vi "LensDistortionCorrectionRpiCam.vi"() -> ()   [LabVIEW 2019]
panel:
  out "Image 2":T1(plugin-control)
  out "Image":T1(plugin-control)
  in  "File Path (Image Calibration 1)":path=path "C:/Users/TTUHEP/Pictures/CalibratedrPiImage.png"
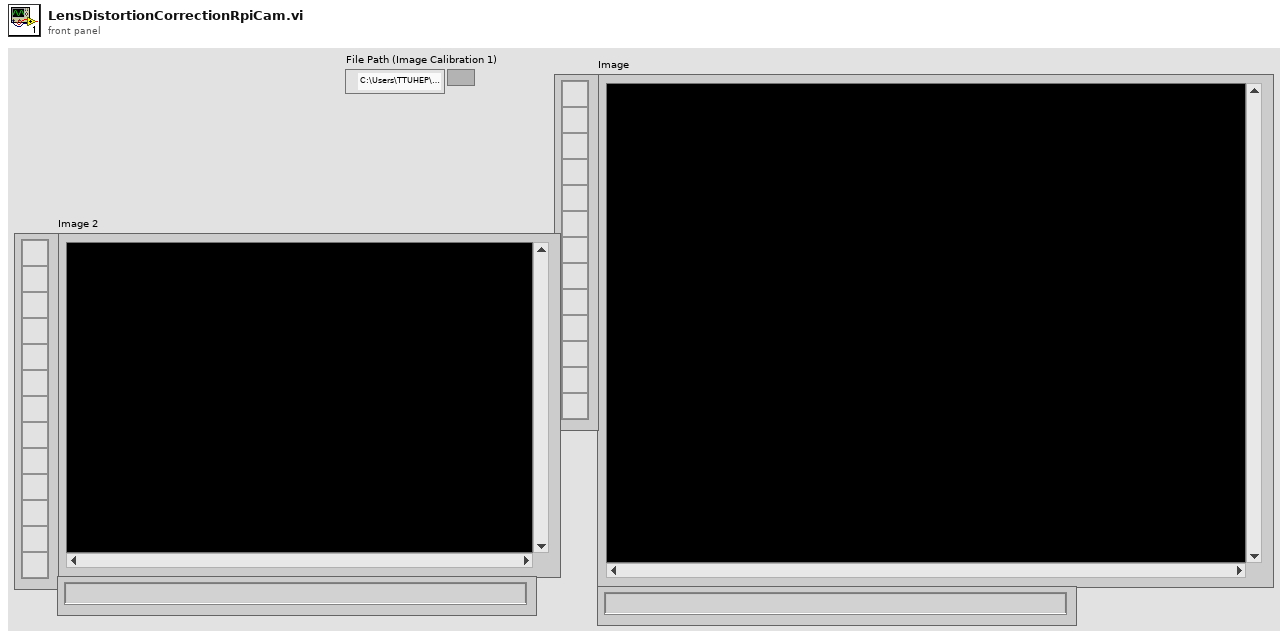
[diagram p1: front panel]
types:
  T1 = typedef "IMAQ Image.ctl" = refnum<image>
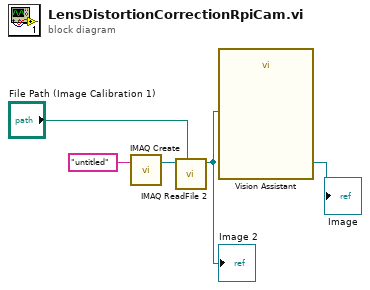
[diagram p0: block diagram]
diagram:
  n1 = call "IMAQ Create"("Image Name"="untitled") -> ("New Image"=w4:T1)  [unwired: 4 in, 1 out]
  n2 = call "IMAQ ReadFile 2"("File Path"="File Path (Image Calibration 1)", "Image"=w4) -> ("Image Out"=w1:T1)  [unwired: 5 in, 4 out]
  "Image 2" <- w1
  n3 = call "Vision Assistant"("Image In"=w1) -> ("Image Out"=→"Image":T1)  [unwired: 25 in, 1 out]
